vi "Stop.vi"(6 "Teller":refnum<class "Teller.lvclass">, 11 "Core Actor in":refnum<class "Core Actor.lvclass">) -> (0 "Error out":errorcluster, 3 "Core Actor out":refnum<class "Core Actor.lvclass">)   [LabVIEW 2025, in "jettl.lvlib" / "Actor.lvlib" / "Core Actor.lvclass"]
uses:
  Core Actor.lvclass
  Teller/Teller/Teller.lvclass
  Core Actor.lvclass/Core Actor.ctl
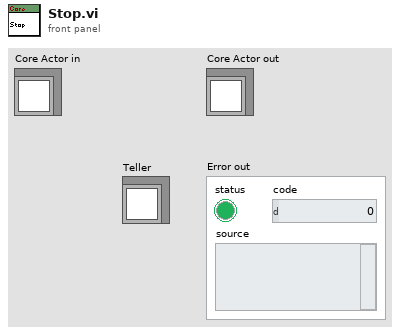
[diagram p1: front panel]
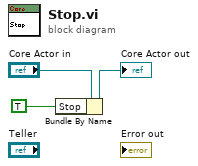
[diagram p0: block diagram]
diagram:
  n1 = Bundle By Name(cluster="Core Actor in", "Stop"=TRUE ("Is Marked For Destroy")) -> (→"Core Actor out":refnum<class "Core Actor.lvclass">)
